vi "Set Parallel Tests Enabled.vi"(8 "error in (no error)":errorcluster, 10 "Parallel tests enabled?":bool, 11 "Configuration Manager In":refnum<class "Configuration Manager.lvclass">) -> (0 "error out":errorcluster, 3 "Configuration Manager Out":refnum<class "Configuration Manager.lvclass">)   [LabVIEW 2020, in "Configuration Manager.lvclass"]
uses:
  Configuration Manager.lvclass
  Configuration Manager.lvclass/Configuration Manager.ctl
  <vilib>/Utility/config.llb/Write Key (Boolean).vi
  <vilib>/Utility/config.llb/NI_LVConfig.lvlib
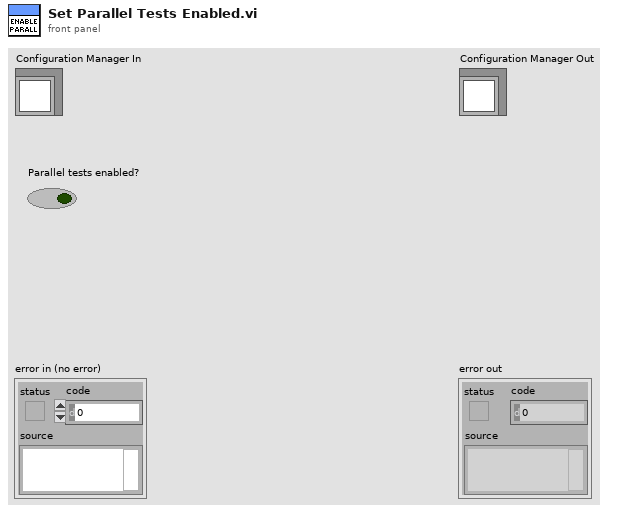
[diagram p1: front panel]
types:
  T1 = typedef "NI_LVConfig.lvlib/Config Data RefNum.ctl" = refnum<k1>
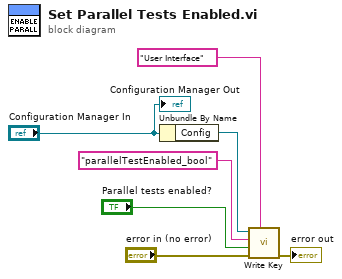
[diagram p0: block diagram]
diagram:
  n1 = Unbundle By Name("Configuration Manager In") -> ("Config"=w6:T1)
  n2 = call-poly <vilib>:"Write Key.vi"("section"="User Interface", "error in (no error)"="error in (no error)", "value"="Parallel tests enabled?", "key"="parallelTestEnabled_bool", "refnum"=w6) -> ("error out"=→"error out":errorcluster)  [unwired: 4 in, 2 out]
  "Configuration Manager Out" <- "Configuration Manager In"
